vi "Recipe_FileLoad.vi"(9 "Recipe_Arr_From_File":string[][](array[string]), 11 "Recipe_Board_Ref":refnum<vi>) -> ()   [LabVIEW 2014]
uses:
  <vilib>/Utility/miscctls.llb/LVBoundsTypeDef.ctl
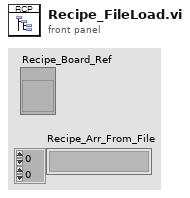
[diagram p1: front panel]
types:
  T1 = typedef "LVBoundsTypeDef.ctl" = cluster{"Width":u32, "Height":u32}
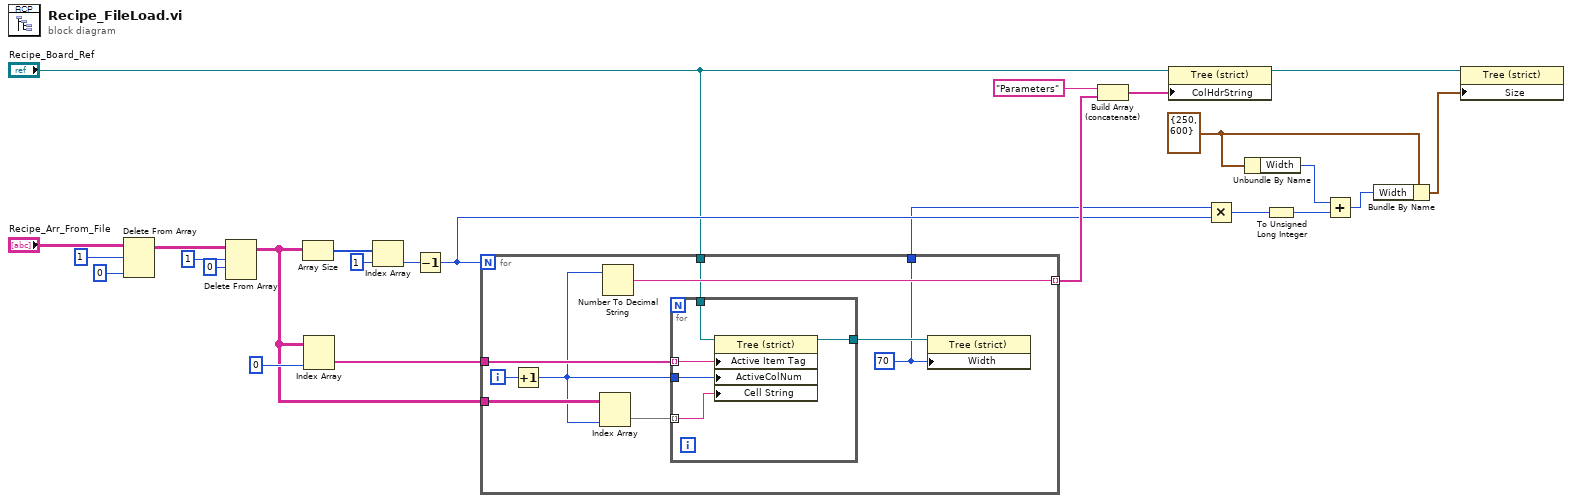
[diagram p0: block diagram]
diagram:
  w8 = T1 {"Width"=250, "Height"=600} ("Size")
  n1 = Delete From Array(array="Recipe_Arr_From_File", length=1, index (col)=0 ("disabled index (col)")) -> (array with subset deleted=w23:string[][])  [unwired: 1 in, 1 out]
  n2 = Delete From Array(array=w23, length=1, index (row)=0) -> (array with subset deleted=w15:string[][])  [unwired: 1 in, 1 out]
  n3 = Array Size(array=w15) -> (size(s)=w19:i32[])
  n4 = Index Array(array=w15, index (col)=0 ("disabled index (col)")) -> (element=w16:string[])  [unwired: 1 in]
  n5 = Index Array(array=w19, index=1) -> (element=w17:i32)
  n6 = Decrement(x=w17) -> (x-1=w9:i32)
  n7 = for {
    N: w9 -> [_]
    tunnel: w16 -> [w34]
    tunnel: w15 -> [w32]
    tunnel: [w29] -> w13 mode=indexing
    tunnel: "Recipe_Board_Ref" -> [w28]
    tunnel: [w26] -> w2
    i -> [w33]
    w26 = 70 ("Active Cell:Cell Size:Width")
    n8 = Increment(x=w33) -> (x+1=w30:i32)
    n9 = Index Array(array=w32, index (col)=w30) -> (element=w31:string[])  [unwired: 1 in]
    n10 = Number To Decimal String(number=w30) -> (decimal integer string=w29:string)  [unwired: 1 in]
    n11 = for {
      tunnel: w34 -> [w39] mode=indexing
      tunnel: w30 -> [w38]
      tunnel: w31 -> [w37] mode=indexing
      tunnel: w28 -> [w36]
      tunnel: [w35] -> w27
      n12 = property on="Property Node" class="Tree (strict)"(reference=w36, "Active Item Tag"=w39, "ActiveColNum"=w38, "Cell String"=w37) -> (reference out=w35:refnum<vi>)  [unwired: 1 in, 1 out]
    }
    n13 = property class="Tree (strict)"(reference=w27, "Width"=w26) -> ()  [unwired: 1 in, 2 out]
  }
  n14 = Build Array (concatenate)("Parameters", w13) -> (w12:string[])
  n15 = property on="Property Node" class="Tree (strict)"(reference="Recipe_Board_Ref", "ColHdrString"=w12) -> (reference out=w10:refnum<vi>)  [unwired: 1 in, 1 out]
  n16 = Multiply(x=w2, y=w9) -> (x*y=w6:i32)
  n17 = Unbundle By Name(w8) -> ("Width"=w5:u32)
  n18 = To Unsigned Long Integer(number=w6) -> (unsigned 32bit integer=w3:u32)
  n19 = Add(x=w5, y=w3) -> (x+y=w4:u32)
  n20 = Bundle By Name(cluster=w8, "Width"=w4) -> (w7:T1)
  n21 = property class="Tree (strict)"(reference=w10, "Size"=w7) -> ()  [unwired: 1 in, 2 out]
